vi "WaitBallKickerSkill.vi"(6 "Role ofRobotThat\nmake the pass":T1=enum."PassKicker", 8 "error in (no error)":errorcluster, 9 "Robot":refnum<class "Robot.lvclass">, 10 "Game":refnum<class "Game.lvclass">, 11 "WaitBallKickerSkill in":refnum<class "WaitBallKickerSkill.lvclass">) -> (0 "error out":errorcluster, 2 "robot out":refnum<class "Robot.lvclass">, 3 "WaitBallKickerSkill out":refnum<class "WaitBallKickerSkill.lvclass">)   [LabVIEW 2024, in "WaitBallKickerSkill.lvclass"]
uses:
  WaitBallKickerSkill.lvclass
  Robot_class/Robot.lvclass
  C:/Users/moise/Documents/GitHub/SSL_AI/Object_class/Object.lvclass
  Game_class/Game.lvclass
  Robot_class/roles.ctl
  Game_class/Game.lvclass/Game.ctl
  Object_class/Object.lvclass/Object.ctl
  Team_class/Team.lvclass/Team.ctl
  Robot_class/Robot.lvclass/Robot.ctl
  Object_class/Read x.vi
  Object_class/Read y.vi
  Game_class/Read BallRef.vi
  Game_class/Read Utilities.lvclass.vi
  Game_class/Read FieldRef.vi
  Game_class/Read OffensiveTeam.vi
  Team_class/Read RobotRef.vi
  Robot_class/Write dest_x.vi
  Robot_class/Write dest_y.vi
  Robot_class/Write dest_orientation.vi
  Ally_class/Ally.lvclass
  C:/Users/moise/Documents/GitHub/SSL_AI/Team_class/Team.lvclass
  Ball_class/Ball.lvclass
  Utilities_class/Utilities.lvclass
  Field_class/Field.lvclass
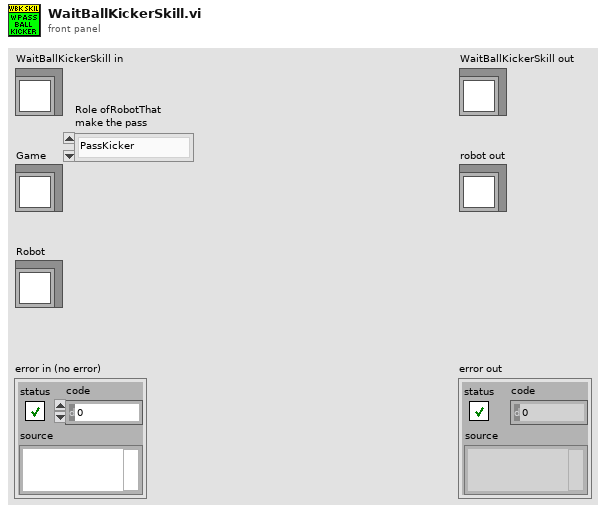
[diagram p1: front panel]
types:
  T1 = typedef "roles.ctl" = enum16{"SimpleBallPlacement", "BallPlacementAllyPasser", "BallPlacementAllyReceiver", "BallPlacementEnemy", "5Robots5th", "PassBestReceiver", "5Robots4th", "5Robots3rd", "5Robots2nd", "5Robots1st", "PassBestRobot", "WaitPass", "ABCThirdKicker", "ABCFirstKicker", "ABCSecondKicker", "Tabler", "TableFinalizer", "PrepareRollToPassRoller", "PrepareRollToPassReceiver", "SimplePassRoll", "SimplePassRollReceiver", "PenaltyDefense", "PreparePassReceiver 2", "PreparePassReceiver 1", "PassObserver", "Timeout", "Goto", "ZigZag", "None", "BallOutOfField", "DefenderArea", "Duelist", "AttackerStop", "FollowAttacker", "KeeperRole", "KickPenalty", "AttackerAimGoal", "AttackerBlock", "Marker", "Halt", "Shoot", "PassKicker", "PassReceiver", "TestRole", "PenaltyAttacker"}
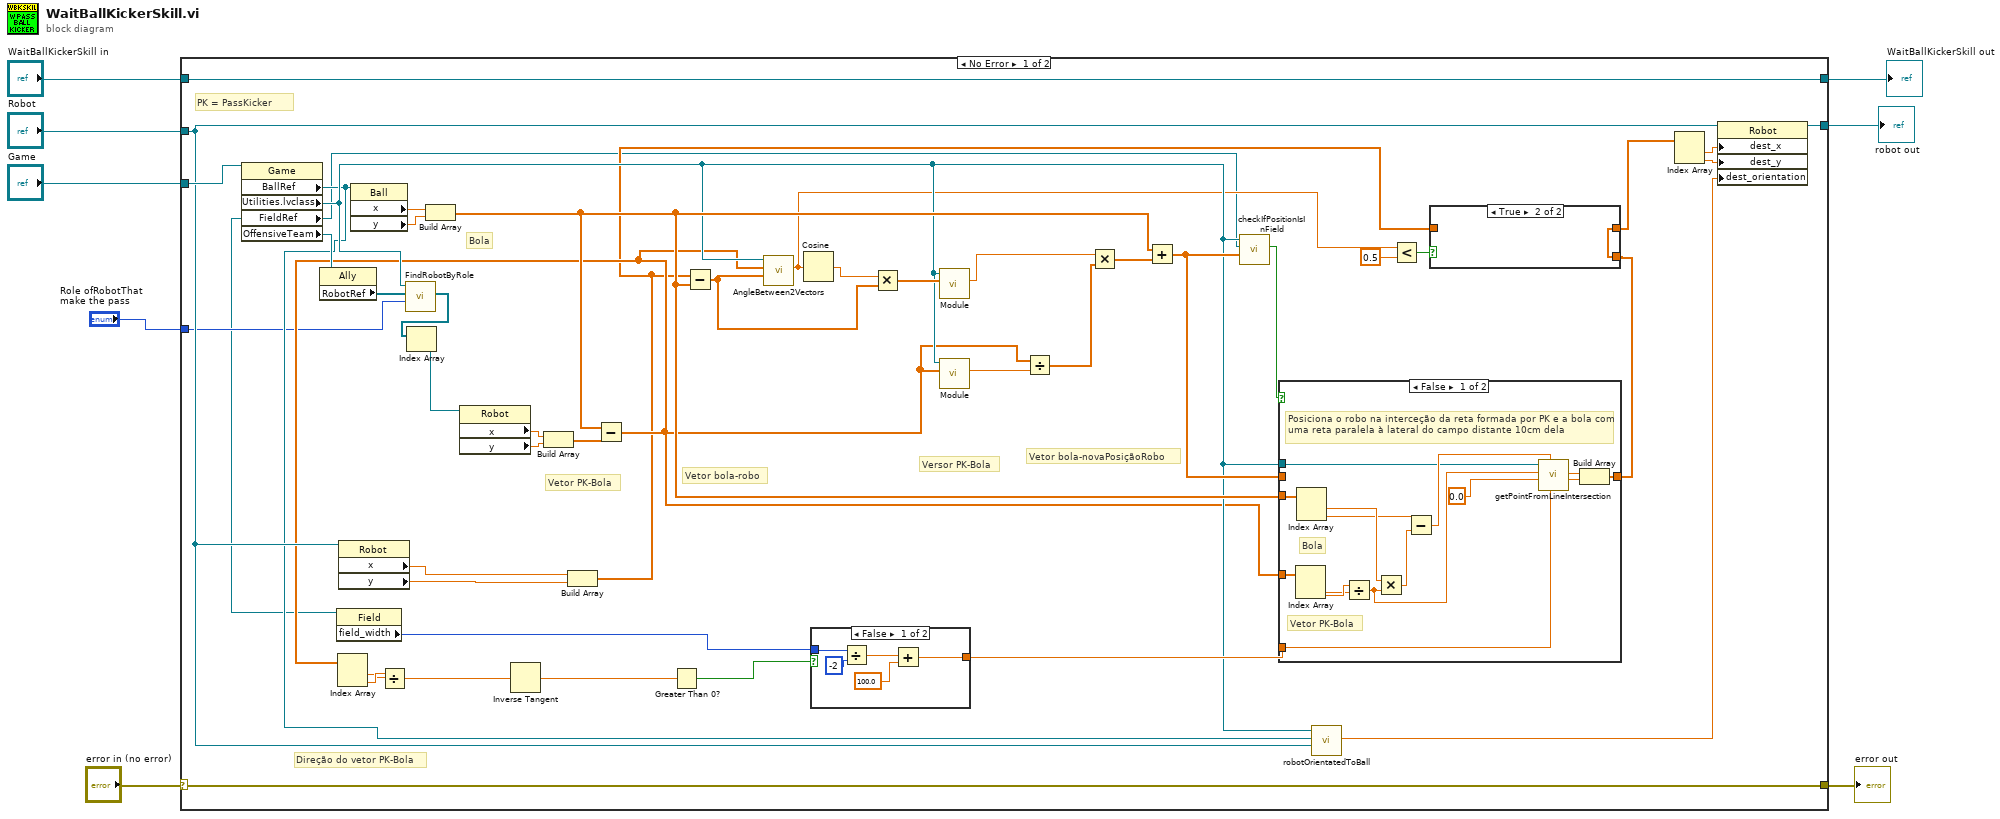
[diagram p0: block diagram]
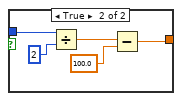
[diagram p3: hidden frame]
diagram:
  n1 = case shown="No Error" "error in (no error)" {
    selector: "error in (no error)" -> [w55 w85]
    tunnel: [w55 w85] -> w7
    tunnel: [w54 w84] -> w5
    tunnel: "WaitBallKickerSkill in" -> [w54 w84]
    tunnel: "Game" -> [w28 _]
    tunnel: "Robot" -> [w27 _]
    tunnel: [w53 _] -> w2
    tunnel: "Role ofRobotThat\nmake the pass" -> [w10 _]
    frame No Error {
      # "Versor PK-Bola"
      # "Bola"
      # "PK = PassKicker"
      # "Vetor PK-Bola"
      # "Direção do vetor PK-Bola"
      # "Vetor bola-novaPosiçãoRobo"
      # "Vetor bola-robo"
      n2 = property class="Game"(reference=w28) -> ("BallRef"=w11:refnum<class "Ball.lvclass">, "Utilities.lvclass"=w22:refnum<class "Utilities.lvclass">, "FieldRef"=w9:refnum<class "Field.lvclass">, "OffensiveTeam"=w36:refnum<class "Ally.lvclass">)  [unwired: 1 in, 2 out]
      n3 = property class="Ally"(reference=w36) -> ("RobotRef"=w35:refnum<class "Robot.lvclass">[])  [unwired: 1 in, 2 out]
      n4 = property class="Field"(reference=w9) -> ("field_width"=w40:i32)  [unwired: 1 in, 2 out]
      n5 = property class="Robot"(reference=w27) -> ("x"=w50:dbl, "y"=w49:dbl)  [unwired: 1 in, 2 out]
      n6 = property class="Ball"(reference=w11) -> ("x"=w52:dbl, "y"=w51:dbl)  [unwired: 1 in, 2 out]
      n7 = call "FindRobotByRole.vi"("role"=w10, "RobotRef"=w35, "Utilities in"=w22) -> ("Robots"=w33:refnum<class "Robot.lvclass">[])  [unwired: 5 in, 3 out]
      n8 = Index Array(array=w33) -> (element=w34:refnum<class "Robot.lvclass">)  [unwired: 1 in]
      n9 = Build Array(w52, w51) -> (w30:dbl[])
      n10 = property class="Robot"(reference=w34) -> ("x"=w32:dbl, "y"=w31:dbl)  [unwired: 1 in, 2 out]
      n11 = Build Array(w32, w31) -> (w18:dbl[])
      n12 = Build Array(w50, w49) -> (w16:dbl[])
      n13 = Subtract(x=w30, y=w18) -> (x-y=w20:dbl[])
      n14 = Index Array(array=w20) -> (element #1=w43:dbl, element #2=w44:dbl)  [unwired: 2 in]
      n15 = Divide(x=w44, y=w43) -> (x/y=w42:dbl)
      n16 = Inverse Tangent(1:w42) -> (0:w29:dbl)
      n17 = Greater Than 0?(x=w29) -> (x > 0?=w41:bool)
      n18 = Subtract(x=w16, y=w30) -> (x-y=w48:dbl[])
      n19 = call "AngleBetween2Vectors.vi"("Array 1"=w48, "Array 2"=w20, "Utilities in"=w22) -> ("angleInRadians(default)"=w12:dbl)  [unwired: 5 in, 3 out]
      n20 = Cosine(x=w12) -> (cos(x)=w47:dbl)
      n21 = case shown="False" w41 {
        tunnel: w40 -> [w61 w67]
        tunnel: [w60 w65] -> w39
        frame False {
          n22 = Divide(x=w61, y=-2) -> (x/y=w59:dbl)
          n23 = Add(x=w59, y=100.0) -> (x+y=w60:dbl)
        }
        frame True {
          n24 = Divide(x=w67, y=2) -> (x/y=w64:dbl)
          n25 = Subtract(x=w64, y=100.0) -> (x-y=w65:dbl)
        }
      }
      n26 = Multiply(x=w47, y=w48) -> (x*y=w25:dbl[])
      n27 = call "Module.vi"("2D vector"=w25, "Utilities in"=w22) -> ("Modulo"=w23:dbl)  [unwired: 7 in, 2 out]
      n28 = call "Module.vi"("2D vector"=w20, "Utilities in"=w22) -> ("Modulo"=w21:dbl)  [unwired: 7 in, 2 out]
      n29 = Divide(x=w20, y=w21) -> (x/y=w19:dbl[])
      n30 = Multiply(x=w23, y=w19) -> (x*y=w24:dbl[])
      n31 = Add(x=w30, y=w24) -> (x+y=w45:dbl[])
      n32 = call "checkIfPositionIsInField.vi"("Position"=w45, "FieldRef"=w9, "Utilities in"=w22) -> ("Position Is In Field?"=w46:bool)  [unwired: 4 in, 4 out]
      n33 = case shown="False" w46 {
        tunnel: w45 -> [_ w83]
        tunnel: [w80 w83] -> w14
        tunnel: w39 -> [w78 _]
        tunnel: w30 -> [w77 _]
        tunnel: w20 -> [w76 _]
        tunnel: w22 -> [w68 _]
        frame False {
          # "Bola"
          # "Vetor PK-Bola"
          # "Posiciona o robo na interceção da reta formada por PK e a bola com uma reta paralela à lateral do campo distante 10cm dela"
          n34 = Index Array(array=w76) -> (element #1=w74:dbl, element #2=w75:dbl)  [unwired: 2 in]
          n35 = Index Array(array=w77) -> (element #1=w73:dbl, element #2=w72:dbl)  [unwired: 2 in]
          n36 = Divide(x=w75, y=w74) -> (x/y=w69:dbl)
          n37 = Multiply(x=w73, y=w69) -> (x*y=w71:dbl)
          n38 = Subtract(x=w72, y=w71) -> (x-y=w70:dbl)
          n39 = call "getPointFromLineIntersection.vi"("b2"=w78, "b1"=w70, "a2"=0.0, "a1"=w69, "Utilities in"=w68) -> ("y_intersection"=w81:dbl, "x_intersection"=w82:dbl)  [unwired: 3 in, 2 out]
          n40 = Build Array(w82, w81) -> (w80:dbl[])
        }
        frame True {
        }
      }
      n41 = call "robotOrientatedToBall.vi"("Robot"=w27, "BallRef"=w11, "Utilities in"=w22) -> ("Orientation"=w26:dbl)  [unwired: 6 in, 2 out]
      n42 = Less?(x=w12, y=0.5) -> (x < y?=w17:bool)
      n43 = case shown="True" w17 {
        tunnel: w16 -> [w56 _]
        tunnel: w14 -> [_ w57]
        tunnel: [w56 w57] -> w13
        frame False {
        }
        frame True {
        }
      }
      n44 = Index Array(array=w13) -> (element #1=w38:dbl, element #2=w37:dbl)  [unwired: 2 in]
      n45 = property class="Robot"(reference=w27, "dest_x"=w38, "dest_y"=w37, "dest_orientation"=w26) -> (reference out=w53:refnum<class "Robot.lvclass">)  [unwired: 1 in, 1 out]
    }
    frame Error {
    }
  }
  "error out" <- w7
  "WaitBallKickerSkill out" <- w5
  "robot out" <- w2
